vi "Build Frame Script Core.vi"(8 "error in (no error)":errorcluster, 10 "Config Array":string[](array[string]), 11 "SPI 3W Pattern Creator in":refnum<class "SPI 3W Pattern Creator.lvclass">) -> (0 "error out":errorcluster, 2 "Pattern Script":string, 3 "SPI 3W Pattern Creator out":refnum<class "SPI 3W Pattern Creator.lvclass">)   [LabVIEW 2018, in "SPI 3W Pattern Creator.lvlib" / "SPI 3W Pattern Creator.lvclass"]
uses:
  SPI 3W Pattern Creator.lvclass
  C:/P4 Workspace/PC Client/Solutions/5g_eap/trunk/1.0/HiSi5GmmWave/Pattern_Gen_Tool/Interfaces/Protocol Interface.lvlibp/Interfaces/Protocol Interface/Protocol Interface.lvclass
  Protocols/SPI Root Pattern Creator.lvlibp/Plugins/SouceCode/SPI_Pattern Creator/SPI Root/Special Frame Type.ctl
  Interfaces/Protocol Interface.lvlibp/Interfaces/Protocol Interface/Read Wait(ms).vi
  Interfaces/Protocol Interface.lvlibp/Interfaces/Protocol Interface/Read Period(ms).vi
  Protocols/SPI Root Pattern Creator.lvlibp/Plugins/SouceCode/SPI_Pattern Creator/SPI Root/SPI Root Pattern Creator.lvclass
  C:/P4 Workspace/PC Client/Solutions/5g_eap/trunk/1.0/HiSi5GmmWave/Pattern_Gen_Tool/Plugins/Protocols/SPI Root Pattern Creator.lvlibp/Plugins/SouceCode/SPI_Pattern Creator/SPI Root/SPI Root Pattern Creator.lvclass
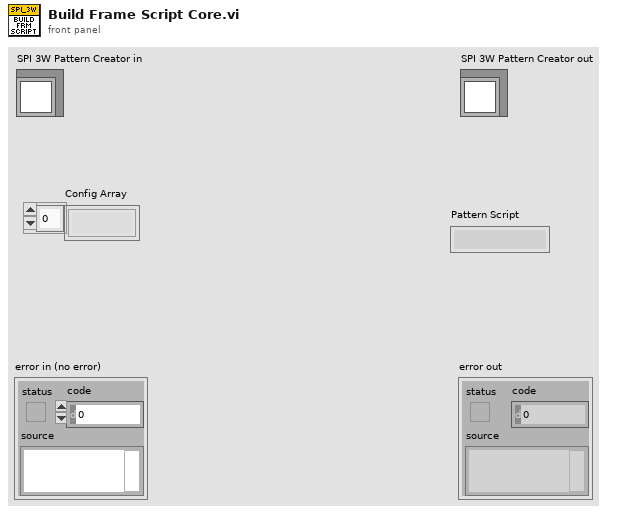
[diagram p1: front panel]
types:
  T1 = typedef "SPI Root Pattern Creator.lvlibp/SPI Root Pattern Creator.lvclass/Special Frame Type.ctl" = enum16{"SPI 4W FRM Start", "SPI 4W Wait", "SPI 4W FRM End", "SPI 4W Write Cmd", "SPI Rd Collect Cmd", "SPI Rd Value Cmd", "SPI 3W FRM Start", "SPI 3W Write Cmd", "SPI 3W FRM End", "SPI 3W Wait", "SPI 3W Rd Cmd"}
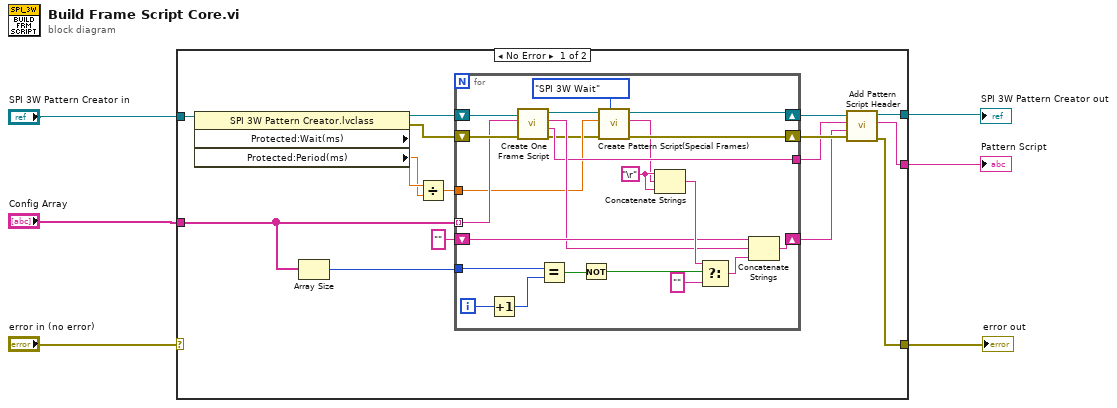
[diagram p0: block diagram]
diagram:
  n1 = case shown="No Error" "error in (no error)" {
    selector: "error in (no error)" -> [_ w46]
    tunnel: "SPI 3W Pattern Creator in" -> [w22 w47]
    tunnel: "Config Array" -> [w16 _]
    tunnel: [w10 w47] -> w3
    tunnel: [w9 w46] -> w2
    tunnel: [w8 _] -> w1
    frame No Error {
      n2 = property class="SPI 3W Pattern Creator.lvclass"(reference=w22) -> (reference out=w17:refnum<class "SPI 3W Pattern Creator.lvclass">, error out=w18:errorcluster, "Protected:Wait(ms)"=w21:dbl, "Protected:Period(ms)"=w20:dbl)  [unwired: 1 in]
      n3 = Array Size(array=w16) -> (size(s)=w15:i32)
      n4 = Divide(x=w21, y=w20) -> (x/y=w19:dbl)
      n5 = for {
        tunnel: w16 -> [w43] mode=indexing
        tunnel: w19 -> [w28]
        shift-right: [w26] -> w13
        shift-left: w18 -> [w44]
        shift-right: [w24] -> w14
        shift-left: w17 -> [w45]
        tunnel: w15 -> [w40]
        shift-right: [w34] -> w12
        shift-left: "" -> [w33]
        tunnel: [w30] -> w11
        i -> [w41]
        w42 = "\r"
        n6 = Increment(x=w41) -> (x+1=w39:i32)
        n7 = call-dynamic "Create One Frame Script.vi"("error in (no error)"=w44, "Config String"=w43, "SPI 3W Pattern Creator in"=w45) -> ("error out"=w27:errorcluster, "Pattern Name out"=w30:string, "Script out"=w32:string, "SPI 3W Pattern Creator out"=w29:refnum<class "SPI 3W Pattern Creator.lvclass">)  [unwired: 5 in]
        n8 = Equal?(x=w40, y=w39) -> (x = y?=w38:bool)
        n9 = Not(x=w38) -> (.not. x?=w37:bool)
        n10 = call "Create Pattern Script(Special Frames).vi"("Special Frame Type"=Special_Frame_Type."SPI 3W Wait", "error in (no error)"=w27, "Num of Timeset"=w28, "SPI Root Pattern Creator in"=w29) -> ("error out"=w26:errorcluster, "String out"=w25:string, "SPI Root Pattern Creator out"=w24:refnum<class "SPI 3W Pattern Creator.lvclass">)  [unwired: 5 in]
        n11 = Concatenate Strings(w42, w25, w42) -> (w36:string)
        n12 = Select(t=w36, s=w37, f="") -> (s? t:f=w31:string)
        n13 = Concatenate Strings(w33, w32, w31) -> (w34:string)
      }
      n14 = call-dynamic "Add Pattern Script Header.vi"("error in (no error)"=w13, "Pattern Script Frame in"=w12, "Pattern Name"=w11, "SPI 3W Pattern Creator in"=w14) -> ("error out"=w9:errorcluster, "Pattern Script All out"=w8:string, "SPI 3W Pattern Creator out"=w10:refnum<class "SPI 3W Pattern Creator.lvclass">)  [unwired: 5 in]
    }
    frame Error {
    }
  }
  "error out" <- w2
  "SPI 3W Pattern Creator out" <- w3
  "Pattern Script" <- w1
